vi "GDFopen2read.vi"(8 "error in":errorcluster, 10 "File path in":path, 11 "GDFv1.x.lvclass in":refnum<class "GDFv1.x.lvclass">) -> (0 "error out":errorcluster, 2 "GDF_header1":T1, 3 "GDFv1.x.lvclass out":refnum<class "GDFv1.x.lvclass">)   [LabVIEW 2016, in "GDF File Reader.lvlib" / "GDFv1.x.lvclass"]
uses:
  GDFv1.x.lvclass
  GdfHeader1.ctl
  <vilib>/Utility/error.llb/DialogType.ctl
  GDFv1.x.lvclass/GDFv1.x.ctl
  GDF File Reader.lvlib
panel:
  # "This VI is a part of BCI Design library, http://www.ru-bci.org \nCopyright © 2020, Sotnikov Peter, All rights reserved. License: GNU GPLv3"
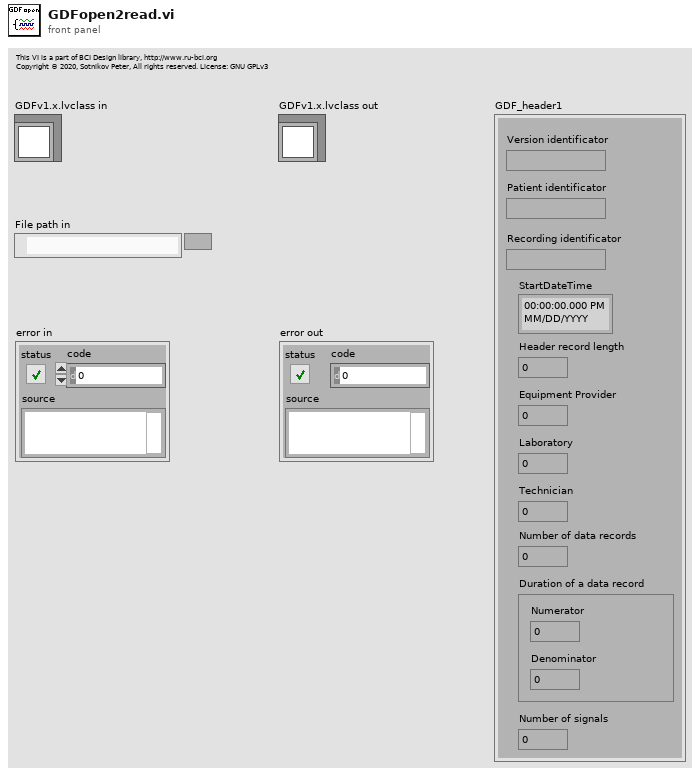
[diagram p1: front panel]
types:
  T1 = typedef "GDF File Reader.lvlib/GdfHeader1.ctl" = cluster{"Version identificator":string, "Patient identificator":string, "Recording identificator":string, "StartDateTime":timestamp, "Header record length":i64, "Equipment Provider":u64, "Laboratory":u64, "Technician":u64, "Number of data records":i64, "Duration of a data record":cluster{"Numerator":u32, "Denominator":u32}, "Number of signals":u32}
  T2 = enum16{"open", "replace", "create", "open or create", "replace or create", "replace or create with confirmation"}
  T3 = enum16{"big-endian, network order", "native, host order", "little-endian"}
  T4 = typedef "DialogType.ctl" = u16
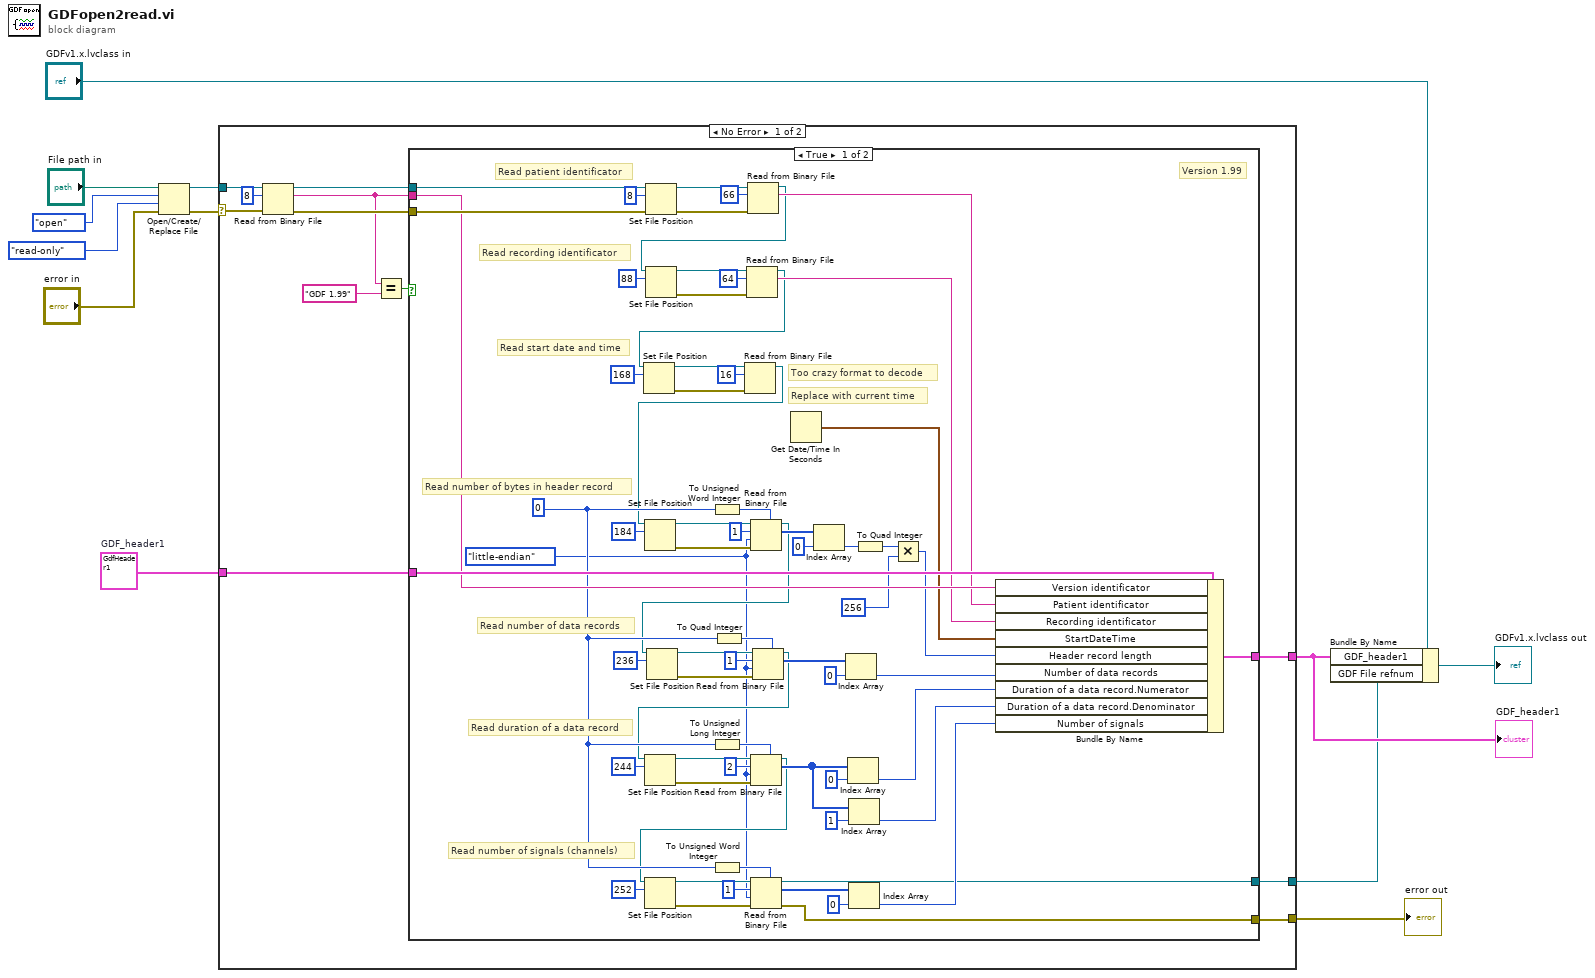
[diagram p0: block diagram]
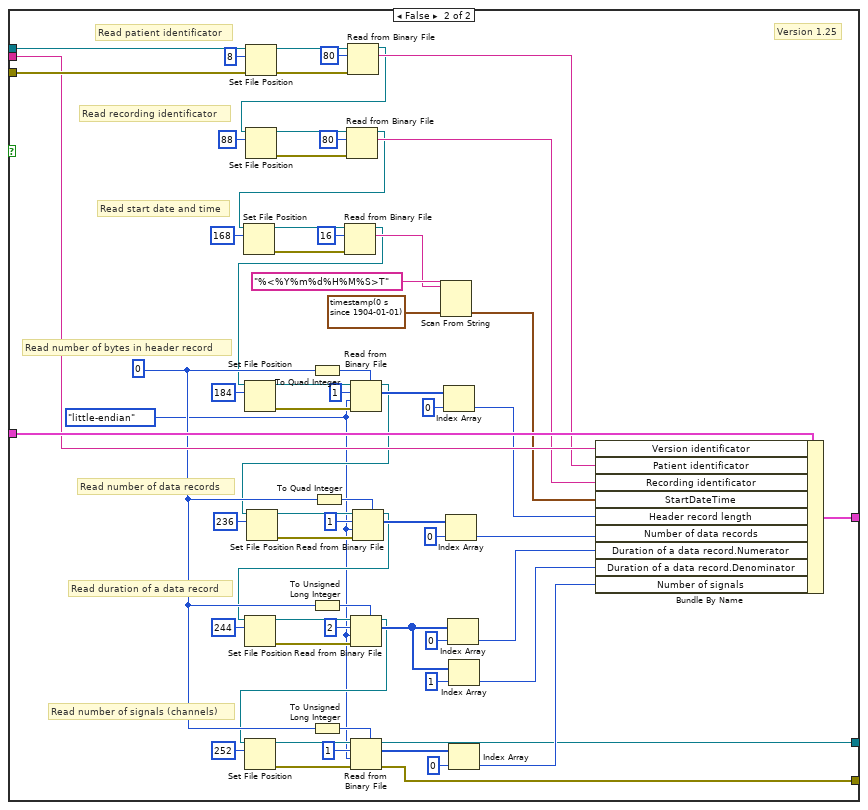
[diagram p2: hidden frame]
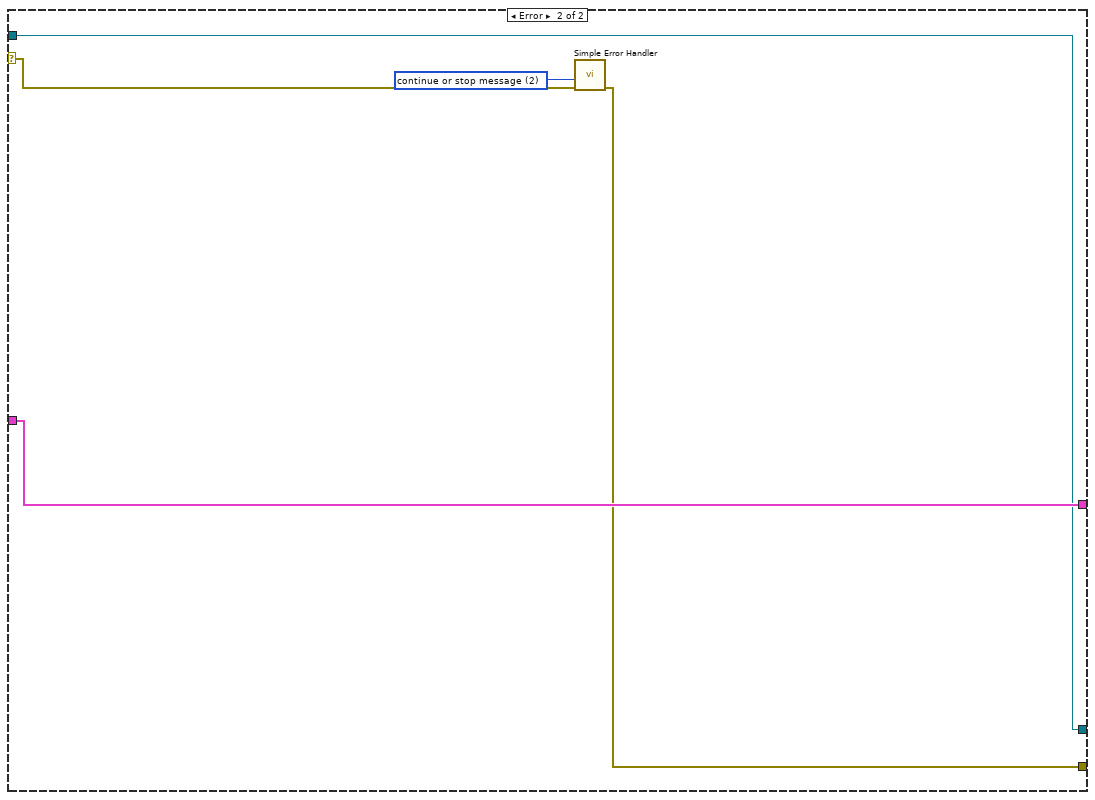
[diagram p3: hidden frame]
diagram:
  w7 = T1 {"Version identificator"="", "Patient identificator"="", "Recording identificator"="", "StartDateTime"=timestamp(0 s since 1904-01-01), "Header record length"=0, "Equipment Provider"=0, "Laboratory"=0, "Technician"=0, "Number of data records"=0, "Duration of a data record"={"Numerator"=0, "Denominator"=0}, "Number of signals"=0}  # GDF_header1
  n1 = Open/Create/Replace File(file path (use dialog)="File path in", error in="error in", operation (0:open)=T2."open", access (0:read/write)=enum16{"read/write", "read-only", "write-only"}."read-only") -> (refnum out=w8:refnum<file>, error out=w9:errorcluster)  [unwired: 2 in, 1 out]
  n2 = case shown="No Error" w9 {
    selector: w9 -> [w24 w161]
    tunnel: w8 -> [w23 w160]
    tunnel: [w18 w163] -> w3
    tunnel: w7 -> [w17 w163]
    tunnel: [w16 w159] -> w5
    tunnel: [w15 w160] -> w2
    frame No Error {
      n3 = Read from Binary File(8:w24, 10:8 ("count (1)"), 11:w23) -> (0:w19:errorcluster, 2:w13:string, 3:w20:refnum<file>)  [unwired: 3 in, 1 out]
      n4 = Equal?(x=w13, y="GDF 1.99" ("regular expression")) -> (x = y?=w21:bool)
      n5 = case shown="True" w21 {
        tunnel: w20 -> [w42 w104]
        tunnel: w19 -> [w91 w158]
        tunnel: w17 -> [w87 w154]
        tunnel: w13 -> [w86 w153]
        tunnel: [w40 w102] -> w18
        tunnel: [w32 w94] -> w16
        tunnel: [w31 w93] -> w15
        frame True {
          w30 = T3."little-endian" ("byte order (0:big-endian, network order)")
          w43 = i64 0 ("offset (in bytes) (0)")
          # "Replace with current time"
          # "Too crazy format to decode"
          # "Version 1.99"
          # "Read number of signals (channels)"
          # "Read duration of a data record"
          # "Read number of data records"
          # "Read number of bytes in header record"
          # "Read start date and time"
          # "Read recording identificator"
          # "Read patient identificator"
          n6 = Set File Position(offset (in bytes) (0)=i64 8, refnum=w42, error in=w91) -> (refnum out=w39:refnum<file>, error out=w89:errorcluster)  [unwired: 1 in]
          n7 = To Unsigned Word Integer(number=w43) -> (unsigned 16bit integer=w72:u16)
          n8 = To Unsigned Long Integer(number=w43) -> (unsigned 32bit integer=w55:u32)
          n9 = To Unsigned Word Integer(number=w43) -> (unsigned 16bit integer=w44:u16)
          n10 = To Quad Integer(1:w43) -> (0:w62:i64)
          n11 = Read from Binary File(8:w89, 10:66 ("count (1)"), 11:w39) -> (2:w81:string, 3:w38:refnum<file>)  [unwired: 3 in, 2 out]
          n12 = Set File Position(offset (in bytes) (0)=i64 88, refnum=w38) -> (refnum out=w82:refnum<file>, error out=w83:errorcluster)  [unwired: 2 in]
          n13 = Read from Binary File(8:w83, 10:64 ("count (1)"), 11:w82) -> (2:w80:string, 3:w37:refnum<file>)  [unwired: 3 in, 2 out]
          n14 = Set File Position(offset (in bytes) (0)=i64 168, refnum=w37) -> (refnum out=w76:refnum<file>, error out=w77:errorcluster)  [unwired: 2 in]
          n15 = Read from Binary File(8:w77, 10:16 ("count (1)"), 11:w76) -> (3:w36:refnum<file>)  [unwired: 3 in, 3 out]
          n16 = Set File Position(offset (in bytes) (0)=i64 184, refnum=w36) -> (refnum out=w74:refnum<file>, error out=w73:errorcluster)  [unwired: 2 in]
          n17 = Read from Binary File(5:w72, 8:w73, 9:w30, 10:1 ("count (1)"), 11:w74) -> (2:w70:u16[], 3:w35:refnum<file>)  [unwired: 1 in, 2 out]
          n18 = Set File Position(offset (in bytes) (0)=i64 236, refnum=w35) -> (refnum out=w67:refnum<file>, error out=w66:errorcluster)  [unwired: 2 in]
          n19 = Read from Binary File(5:w62, 8:w66, 9:w30, 10:1 ("count (1)"), 11:w67) -> (2:w64:i64[], 3:w34:refnum<file>)  [unwired: 1 in, 2 out]
          n20 = Set File Position(offset (in bytes) (0)=i64 244, refnum=w34) -> (refnum out=w59:refnum<file>, error out=w58:errorcluster)  [unwired: 2 in]
          n21 = Read from Binary File(5:w55, 8:w58, 9:w30, 10:2 ("count (1)"), 11:w59) -> (2:w53:u32[], 3:w33:refnum<file>)  [unwired: 1 in, 2 out]
          n22 = Set File Position(offset (in bytes) (0)=i64 252, refnum=w33) -> (refnum out=w49:refnum<file>, error out=w48:errorcluster)  [unwired: 2 in]
          n23 = Read from Binary File(5:w44, 8:w48, 9:w30, 10:1 ("count (1)"), 11:w49) -> (0:w32:errorcluster, 2:w46:u16[], 3:w31:refnum<file>)  [unwired: 1 in, 1 out]
          n24 = Get Date/Time In Seconds() -> (seconds since 1Jan1904=w29:timestamp)
          n25 = Index Array(array=w70, index=0) -> (element=w26:u16)
          n26 = Index Array(array=w64, index=0) -> (element=w61:i64)
          n27 = Index Array(array=w53, index=0) -> (element=w52:u32)
          n28 = Index Array(array=w53, index=1) -> (element=w51:u32)
          n29 = Index Array(array=w46, index=0) -> (element=w41:u16)
          n30 = To Quad Integer(1:w26) -> (0:w27:i64)
          n31 = Multiply(x=w27, y=i64 256) -> (x*y=w28:i64)
          n32 = Bundle By Name(cluster=w87, "Version identificator"=w86, "Patient identificator"=w81, "Recording identificator"=w80, "StartDateTime"=w29, "Header record length"=w28, "Number of data records"=w61, "Duration of a data record.Numerator"=w52, "Duration of a data record.Denominator"=w51, "Number of signals"=w41) -> (w40:T1)
        }
        frame False {
          w92 = T3."little-endian" ("byte order (0:big-endian, network order)")
          w105 = i64 0 ("offset (in bytes) (0)")
          # "Version 1.25"
          # "Read number of signals (channels)"
          # "Read duration of a data record"
          # "Read number of data records"
          # "Read number of bytes in header record"
          # "Read start date and time"
          # "Read recording identificator"
          # "Read patient identificator"
          n33 = Set File Position(offset (in bytes) (0)=i64 8, refnum=w104, error in=w158) -> (refnum out=w101:refnum<file>, error out=w156:errorcluster)  [unwired: 1 in]
          n34 = To Quad Integer(1:w105) -> (0:w136:i64)
          n35 = To Unsigned Long Integer(number=w105) -> (unsigned 32bit integer=w117:u32)
          n36 = To Unsigned Long Integer(number=w105) -> (unsigned 32bit integer=w106:u32)
          n37 = To Quad Integer(1:w105) -> (0:w124:i64)
          n38 = Read from Binary File(8:w156, 10:80 ("count (1)"), 11:w101) -> (2:w148:string, 3:w100:refnum<file>)  [unwired: 3 in, 2 out]
          n39 = Set File Position(offset (in bytes) (0)=i64 88, refnum=w100) -> (refnum out=w149:refnum<file>, error out=w150:errorcluster)  [unwired: 2 in]
          n40 = Read from Binary File(8:w150, 10:80 ("count (1)"), 11:w149) -> (2:w147:string, 3:w99:refnum<file>)  [unwired: 3 in, 2 out]
          n41 = Set File Position(offset (in bytes) (0)=i64 168, refnum=w99) -> (refnum out=w143:refnum<file>, error out=w144:errorcluster)  [unwired: 2 in]
          n42 = Read from Binary File(8:w144, 10:16 ("count (1)"), 11:w143) -> (2:w140:string, 3:w98:refnum<file>)  [unwired: 3 in, 2 out]
          n43 = Set File Position(offset (in bytes) (0)=i64 184, refnum=w98) -> (refnum out=w138:refnum<file>, error out=w137:errorcluster)  [unwired: 2 in]
          n44 = Read from Binary File(5:w136, 8:w137, 9:w92, 10:1 ("count (1)"), 11:w138) -> (2:w133:i64[], 3:w97:refnum<file>)  [unwired: 1 in, 2 out]
          n45 = Set File Position(offset (in bytes) (0)=i64 236, refnum=w97) -> (refnum out=w129:refnum<file>, error out=w128:errorcluster)  [unwired: 2 in]
          n46 = Read from Binary File(5:w124, 8:w128, 9:w92, 10:1 ("count (1)"), 11:w129) -> (2:w126:i64[], 3:w96:refnum<file>)  [unwired: 1 in, 2 out]
          n47 = Set File Position(offset (in bytes) (0)=i64 244, refnum=w96) -> (refnum out=w121:refnum<file>, error out=w120:errorcluster)  [unwired: 2 in]
          n48 = Read from Binary File(5:w117, 8:w120, 9:w92, 10:2 ("count (1)"), 11:w121) -> (2:w115:u32[], 3:w95:refnum<file>)  [unwired: 1 in, 2 out]
          n49 = Set File Position(offset (in bytes) (0)=i64 252, refnum=w95) -> (refnum out=w111:refnum<file>, error out=w110:errorcluster)  [unwired: 2 in]
          n50 = Read from Binary File(5:w106, 8:w110, 9:w92, 10:1 ("count (1)"), 11:w111) -> (0:w94:errorcluster, 2:w108:u32[], 3:w93:refnum<file>)  [unwired: 1 in, 1 out]
          n51 = Scan From String(format string="%<%Y%m%d%H%M%S>T", input string=w140, default 1=timestamp(0 s since 1904-01-01) ("default value 1")) -> (output 1=w134:timestamp)  [unwired: 2 in, 3 out]
          n52 = Index Array(array=w133, index=0) -> (element=w131:i64)
          n53 = Index Array(array=w126, index=0) -> (element=w123:i64)
          n54 = Index Array(array=w115, index=0) -> (element=w114:u32)
          n55 = Index Array(array=w115, index=1) -> (element=w113:u32)
          n56 = Index Array(array=w108, index=0) -> (element=w103:u32)
          n57 = Bundle By Name(cluster=w154, "Version identificator"=w153, "Patient identificator"=w148, "Recording identificator"=w147, "StartDateTime"=w134, "Header record length"=w131, "Number of data records"=w123, "Duration of a data record.Numerator"=w114, "Duration of a data record.Denominator"=w113, "Number of signals"=w103) -> (w102:T1)
        }
      }
    }
    frame Error {
      w162 = T4 2 items=["no dialog", "OK message", "continue or stop message", "OK message + warnings", "continue/stop + warnings"] ("type of dialog (OK msg:1)")
      n58 = call <vilib>:"Simple Error Handler.vi"("type of dialog (OK msg:1)"=w162, "error in (no error)"=w161) -> ("error out"=w159:errorcluster)  [unwired: 3 in, 4 out]
    }
  }
  "error out" <- w5
  "GDF_header1" <- w3
  n59 = Bundle By Name(cluster="GDFv1.x.lvclass in", "GDF_header1"=w3, "GDF File refnum"=w2) -> (→"GDFv1.x.lvclass out":refnum<class "GDFv1.x.lvclass">)
